vi "Read S24.vi"(0 "I2C In":refnum<class "I2C.lvclass">, 1 "Slave Address":u8, 5 "Register":u32, 11 "Error In":errorcluster, 12 "Register Size":T2, 13 "Byte Order":T1) -> (4 "I2C Out":refnum<class "I2C.lvclass">, 6 "Value":i32, 15 "Error Out":errorcluster)   [LabVIEW 2020, in "lv_i2c_hal.lvlib" / "I2C.lvclass"]
uses:
  I2C.lvclass
  Register Address Size.ctl
  Byte Order.ctl
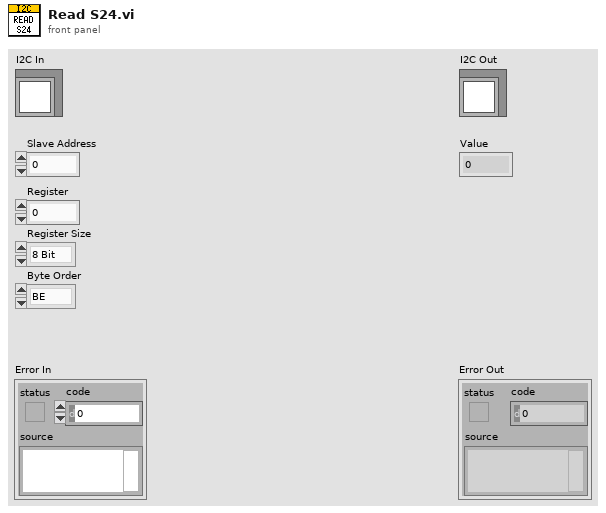
[diagram p1: front panel]
types:
  T1 = typedef "lv_i2c_hal.lvlib/I2C.lvclass/Byte Order.ctl" = enum16{"BE", "LE"}
  T2 = typedef "lv_i2c_hal.lvlib/I2C.lvclass/Register Address Size.ctl" = enum16{"8 Bit", "16 Bit", "24 Bit", "32 Bit"}
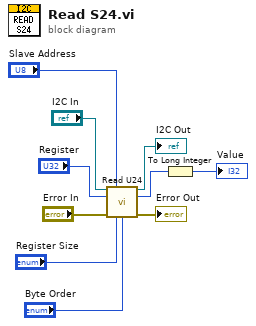
[diagram p0: block diagram]
diagram:
  n1 = call "Read U24.vi"("I2C In"="I2C In", "Slave Address"="Slave Address", "Register"="Register", "Error In"="Error In", "Register Size"="Register Size", "Byte Order"="Byte Order") -> ("I2C Out"=→"I2C Out":refnum<class "I2C.lvclass">, "Value"=w2:u32, "Error Out"=→"Error Out":errorcluster)  [unwired: 7 in]
  n2 = To Long Integer(number=w2) -> (32bit integer=→"Value":i32)
